vi "IsProjectItemPublic.vi"(10 "ProjectItem Refnum":refnum<vi>) -> (2 "Is Public":bool)   [LabVIEW 2019, in "LVUnitTestBuilder.lvclass"]
doc: "Returns true if the specified project item is in public scope."
uses:
  LVUnitTestBuilder.lvclass
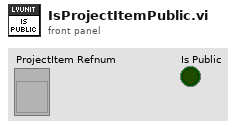
[diagram p1: front panel]
types:
  T1 = enum32{"invalid scope", "public", "private", "protected", "community"}
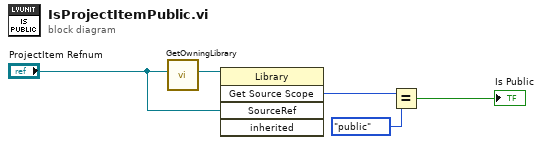
[diagram p0: block diagram]
diagram:
  n1 = call "GetOwningLibrary.vi"("Parent"="ProjectItem Refnum") -> ("Owner"=w5:refnum<vi>)  [unwired: 10 in]
  n2 = invoke class="Library" method="Get Source Scope"(reference=w5, "SourceRef"="ProjectItem Refnum") -> ("GetSourceScope"=w2:T1)  [unwired: 3 in, 4 out]
  n3 = Equal?(x=w2, y=T1."public") -> (x = y?=→"Is Public":bool)
